vi "AvalableLogFiles.vi"(0 "path":path, 11 "error in (no error)":errorcluster) -> (4 "FilesInfo":string[][](array[string]), 15 "error out":errorcluster)   [LabVIEW 2017, in "AppStateMachine runtime.lvclass"]
uses:
  AppStateMachine runtime.lvclass
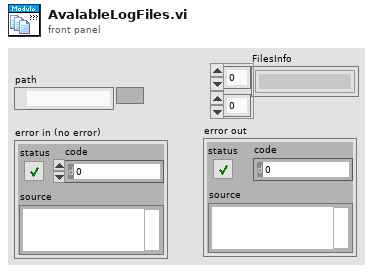
[diagram p1: front panel]
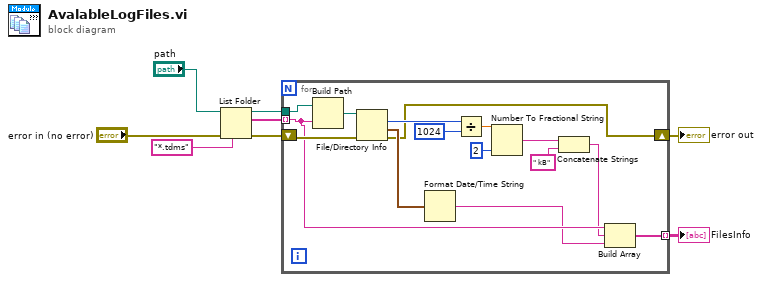
[diagram p0: block diagram]
diagram:
  n1 = List Folder(path="path", pattern="*.tdms", error in="error in (no error)") -> (path out=w5:path, filenames=w4:string[], error out=w3:errorcluster)  [unwired: 1 in, 1 out]
  n2 = for {
    tunnel: w5 -> [w23]
    tunnel: w4 -> [w12] mode=indexing
    shift-right: [w13] -> w2
    shift-left: w3 -> [w21]
    tunnel: [w9] -> w1 mode=indexing
    n3 = Build Path(base path=w23, name or relative path=w12) -> (appended path=w22:path)
    n4 = File/Directory Info(path=w22, error in=w21) -> (size=w20:i64, last mod=w14:timestamp, error out=w13:errorcluster)  [unwired: 4 out]
    n5 = Format Date/Time String(seconds (now)=w14) -> (date/time string=w10:string)  [unwired: 2 in]
    n6 = Divide(x=w20, y=i64 1024) -> (x/y=w18:dbl)
    n7 = Number To Fractional String(number=w18, precision (6)=i16 2) -> (F-format string=w16:string)  [unwired: 2 in]
    n8 = Concatenate Strings(w16, " kB" ("string")) -> (w11:string)
    n9 = Build Array(w12, w11, w10) -> (w9:string[])
  }
  "error out" <- w2
  "FilesInfo" <- w1
